vi "CSM - Mermaid - DebugTool.vi"() -> ()   [LabVIEW 2020]
doc: "Show CSM relationship Graph with mermaid"
uses:
  <vilib>/sklein/WebView2 XControl/WebView2 XControl/WebView2 Control.xctl
  <userlib>/_NEVSTOP/Communicable State Machine(CSM)/_Support/Typedef/_CSM_GlobalLog_MSG.ctl
  <userlib>/_NEVSTOP/Communicable State Machine(CSM)/_Support/Typedef/_CSM_Response Source Message.ctl
  <userlib>/_NEVSTOP/Communicable State Machine(CSM)/_Support/Typedef/_CSM_GlobalLog_MSG_TYPE.ctl
  <userlib>/_NEVSTOP/Communicable State Machine(CSM)/AdvanceAPI/CSM - Convert Error to Argument.vi
  <userlib>/_NEVSTOP/Communicable State Machine(CSM)/_Support/GlobalEvent/GEvt-Generate with Rule Check.vi
  <userlib>/_NEVSTOP/Communicable State Machine(CSM)/_Support/GlobalEvent/Cache-GEvt Refs.vi
  <userlib>/_NEVSTOP/Communicable State Machine(CSM)/AdvanceAPI/CSM - Make String Arguments Safe.vi
  <userlib>/_NEVSTOP/Communicable State Machine(CSM)/_Support/ChangeFlag/FlagInstance-GEvt Refs.vi
  <userlib>/_NEVSTOP/Communicable State Machine(CSM)/AdvanceAPI/CSM - Keywords.vi
  <userlib>/_NEVSTOP/Communicable State Machine(CSM)/_Support/ChangeFlag/ChangeFlag-Read.vi
  <userlib>/_NEVSTOP/Communicable State Machine(CSM)/_Polymophic/Add State(s) to Queue By BOOL(Element).vi
  <userlib>/_NEVSTOP/Communicable State Machine(CSM)/_Support/ChangeFlag/ChangeFlagDB.vi
  <userlib>/_NEVSTOP/Communicable State Machine(CSM)/_Support/GlobalEvent/FGV-GlobalEventRef(lvlibp).vi
  <userlib>/_NEVSTOP/Communicable State Machine(CSM)/_Support/GlobalEvent/FGV-GlobalEventQueues(lvlibp).vi
  <userlib>/_NEVSTOP/Communicable State Machine(CSM)/_Support/GlobalEvent/GEvt-Valid Subscribers.vi
  <userlib>/_NEVSTOP/Communicable State Machine(CSM)/_Support/GlobalEvent/LogFilter/LogFilter - Check.vi
  <userlib>/_NEVSTOP/Communicable State Machine(CSM)/_csmHelper/API/Create From VI Reference.vi
  <userlib>/_NEVSTOP/Communicable State Machine(CSM)/_csmHelper/API/Destroy.vi
  <userlib>/_NEVSTOP/Communicable State Machine(CSM)/_Support/GlobalEvent/LogFilter/LogFilter.lvclass
  <userlib>/_NEVSTOP/Communicable State Machine(CSM)/Communicable State Machine.lvlib
  _support/CSM Mermaid Support.lvlib
  <userlib>/_NEVSTOP/Communicable State Machine(CSM)/_csmHelper/CSM-Helper.lvclass
  <userlib>/_NEVSTOP/Communicable State Machine(CSM)/_tool/_file/csm-file-support.lvlib
  <userlib>/_NEVSTOP/Communicable State Machine(CSM)/_tool/_ui/csm-ui-support.lvlib
panel:
  in  "CSM":string(combo)
  in  "Search Button":bool
  in  "Draw Mermaid":bool
  in  "Type":T1(ring)
  in  "Tab":T2(tab)
  out "Broadcast Registry":string[][](table)
  out "mermaid string":string
  in  "WebView2 Control":string(xcontrol)
  # "https://mermaid.live/"
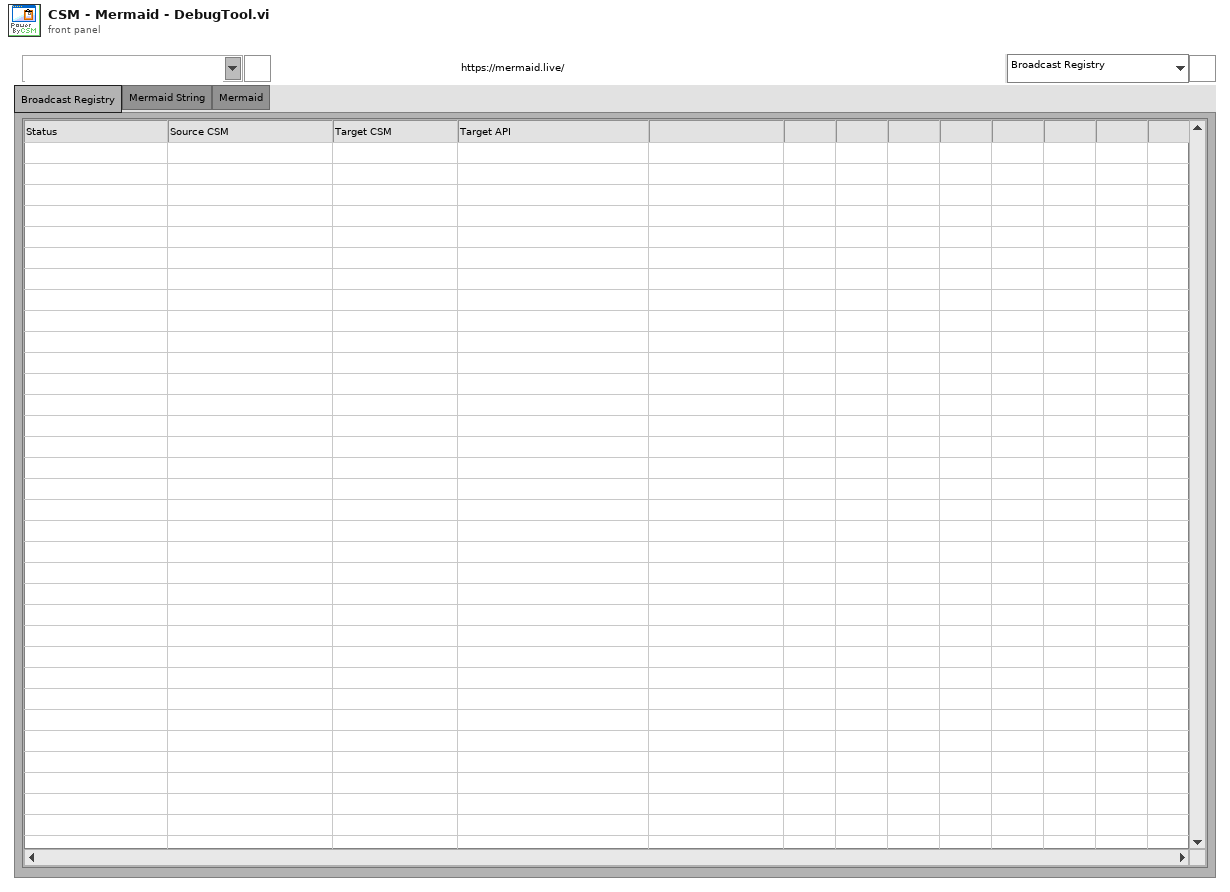
[diagram p1: front panel]
types:
  T1 = enum16{"Broadcast Registry", "CSM Interface", "CSM All Interfaces"}
  T2 = enum32{"Broadcast Registry", "Mermaid String", "Mermaid"}
  T3 = typedef "Communicable State Machine.lvlib/_CSM_GlobalLog_MSG.ctl" = cluster{"Name (\"\" to Use UUID)":string, "Current State":string, "Arguments":string, "Source Message":T4, "Source Module":string, "Complete(T)/Start(F)":bool, "LogType":T5, "Time Stamp":timestamp}
  T4 = typedef "Communicable State Machine.lvlib/_CSM_Response Source Message.ctl" = cluster{"‘State":string, "’Arguments":string, "’Error":errorcluster}
  T5 = typedef "Communicable State Machine.lvlib/_CSM_GlobalLog_MSG_TYPE.ctl" = enum16{"User Log", "State Change", "Status", "Interrupt", "Register", "Unregister", "Error Log", "Module Created", "Module Destroyed", "Async Message", "No-Rep Async Message", "Sync Message"}
  T6 = enum32{"Broadcast Registry", "Mermaid String", "Mermaid", "Error History"}
  T7 = enum32{"Invalid", "Standard", "Closed", "Hidden", "Minimized", "Maximized"}
  T8 = enum32{"invalid app kind", "Development System", "Run Time System", "Student Edition", "Embedded LabVIEW", "Evaluation", "Custom"}
  T9 = cluster{"Shift":bool, "Ctrl":bool, "Alt":bool, "Cmd":bool, "Opt":bool}
  T10 = cluster{"Core":cluster{"Current VI Reference":refnum<vi>, "Close Panel on Exit?":bool}, "Toolbar.Advance":refnum<vi>[], "LoggerWatchDogQueue":refnum<queue>, "LogFile":path, "Mermaid":cluster{"Template":string, "output path":path, "string":string}}
  T11 = cluster{"Template":string, "output path":path, "string":string}
  T12 = cluster{"Current VI Reference":refnum<vi>, "Close Panel on Exit?":bool}
  T13 = cluster{"Status":string, "Source CSM":string, "Target CSM":string, "Target API":string}[]
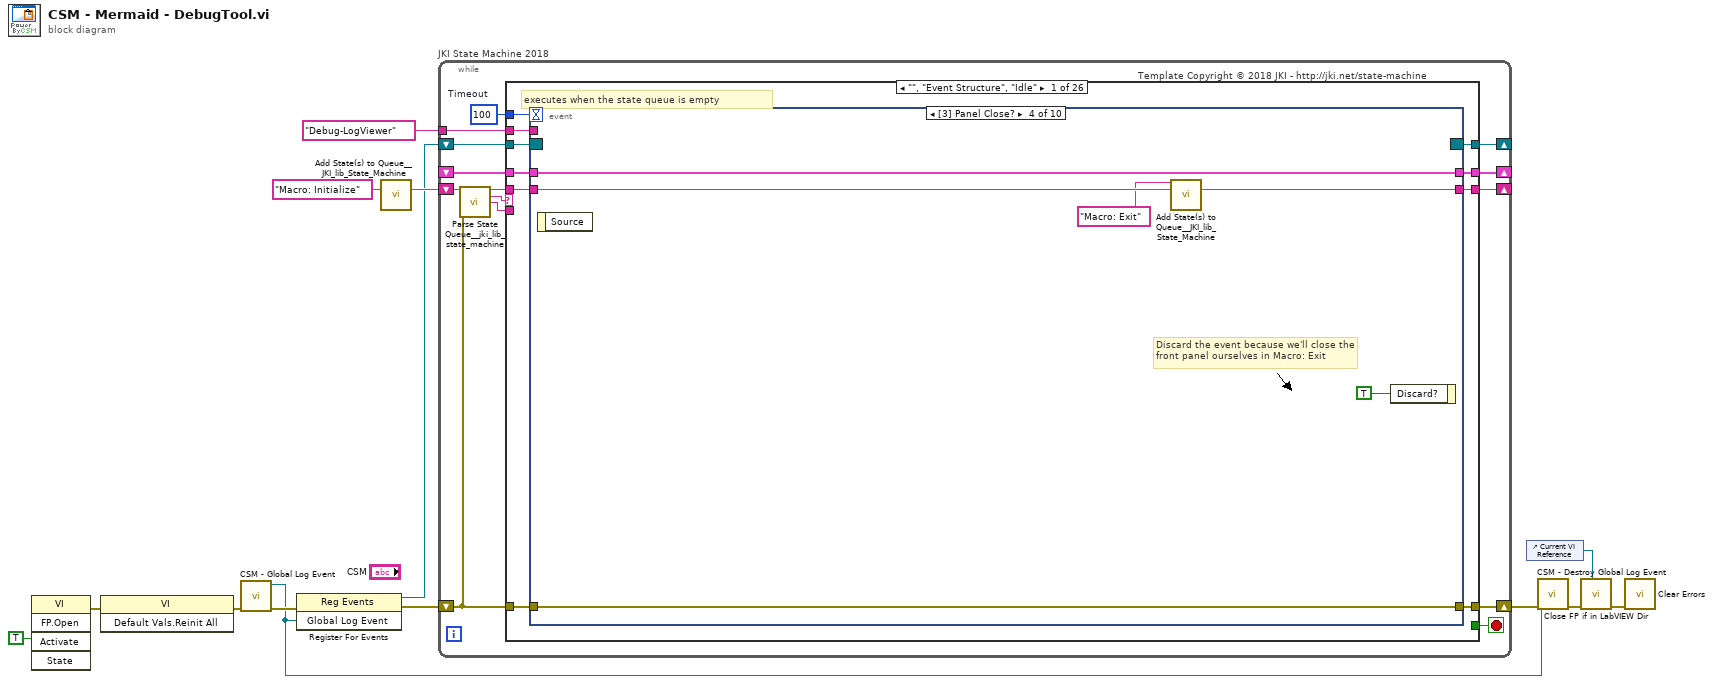
[diagram p0: block diagram]
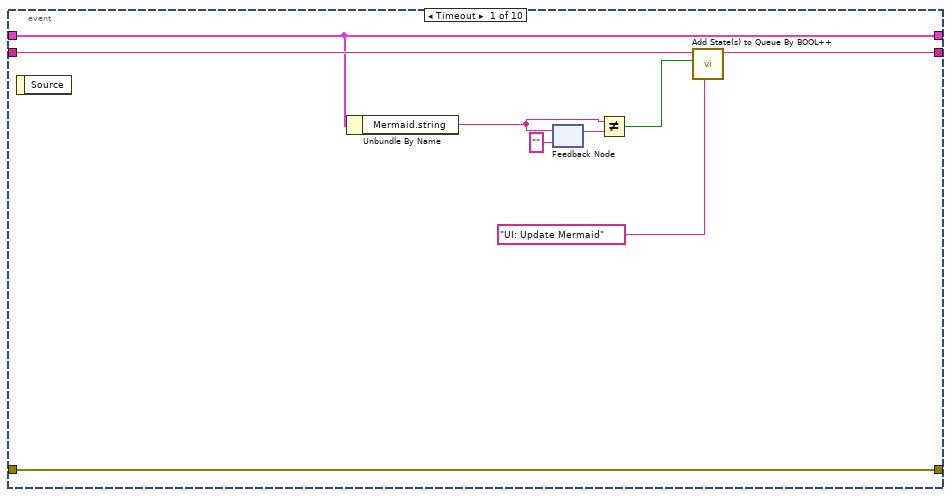
[diagram p2: hidden frame]
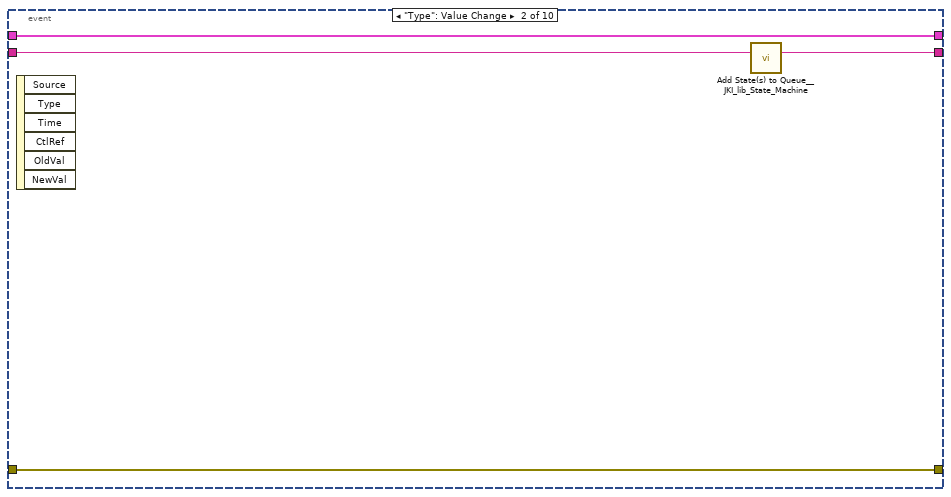
[diagram p3: hidden frame]
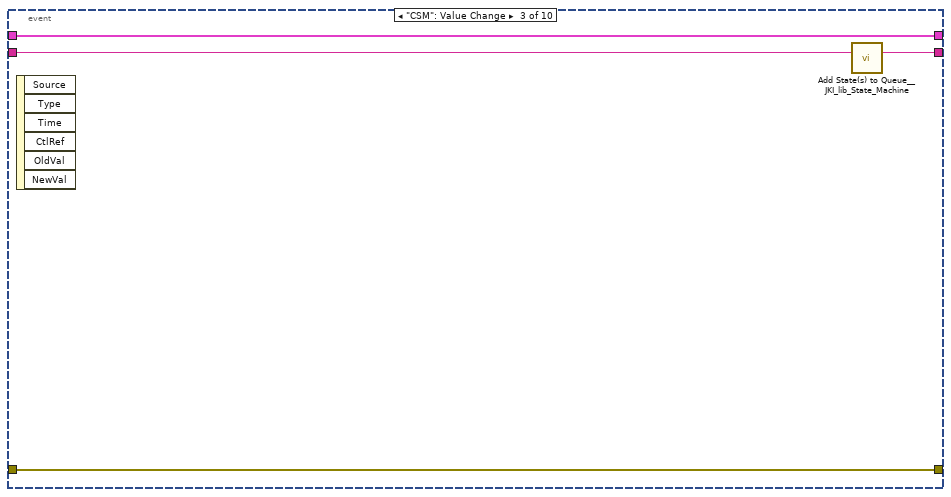
[diagram p4: hidden frame]
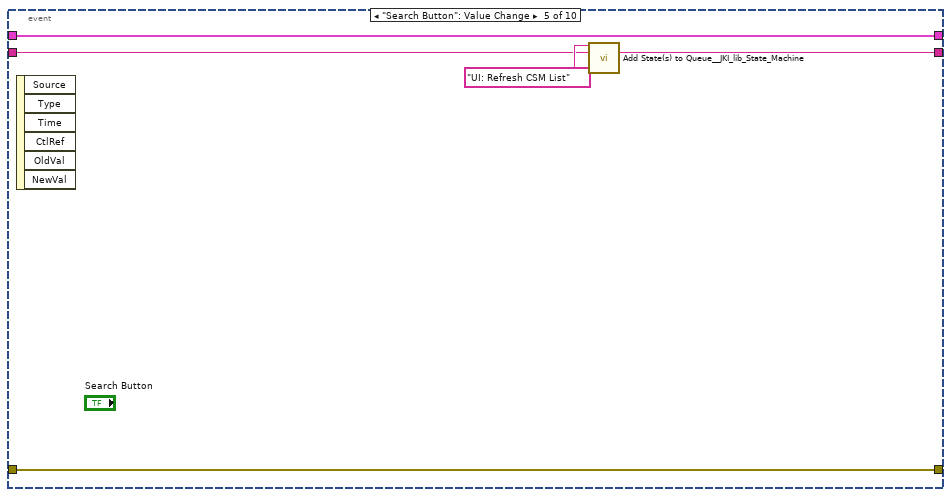
[diagram p5: hidden frame]
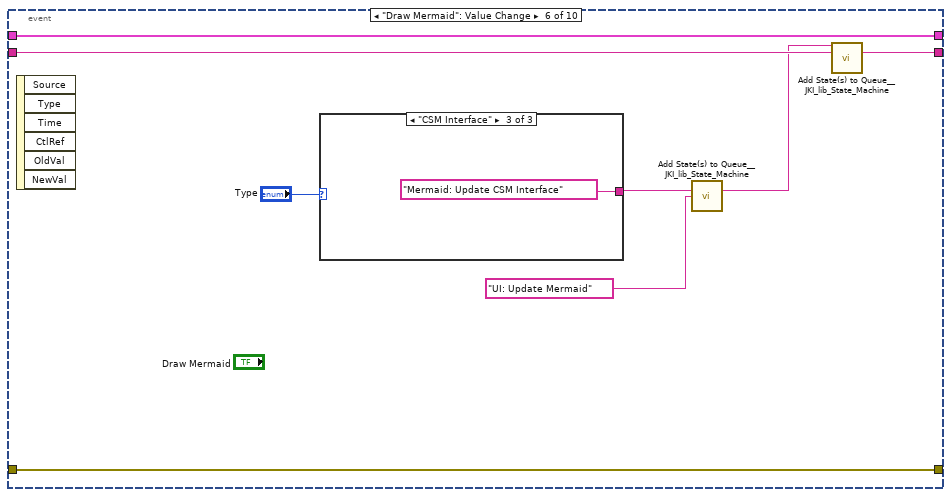
[diagram p6: hidden frame]
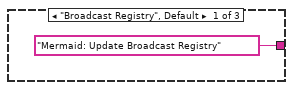
[diagram p7: hidden frame]
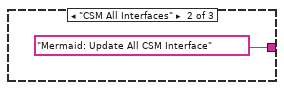
[diagram p8: hidden frame]
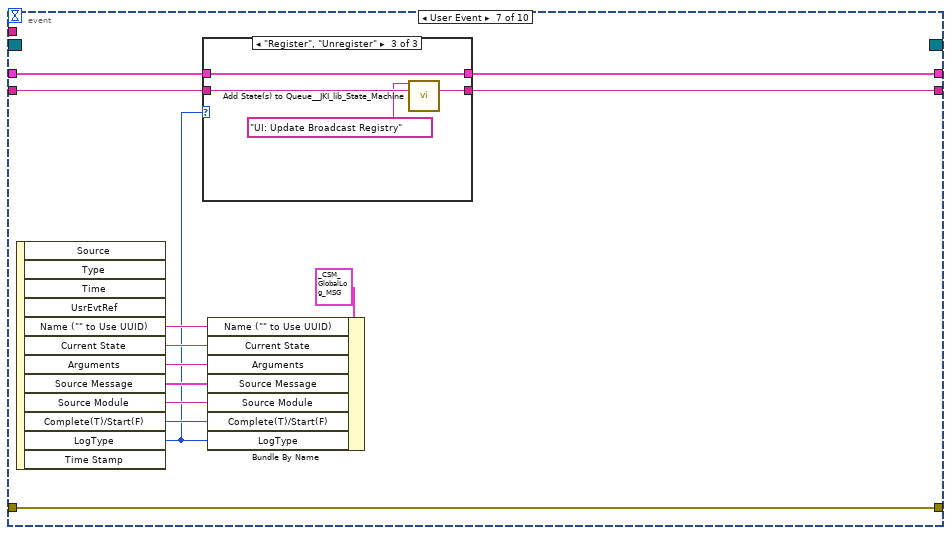
[diagram p9: hidden frame]
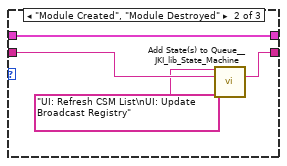
[diagram p11: hidden frame]
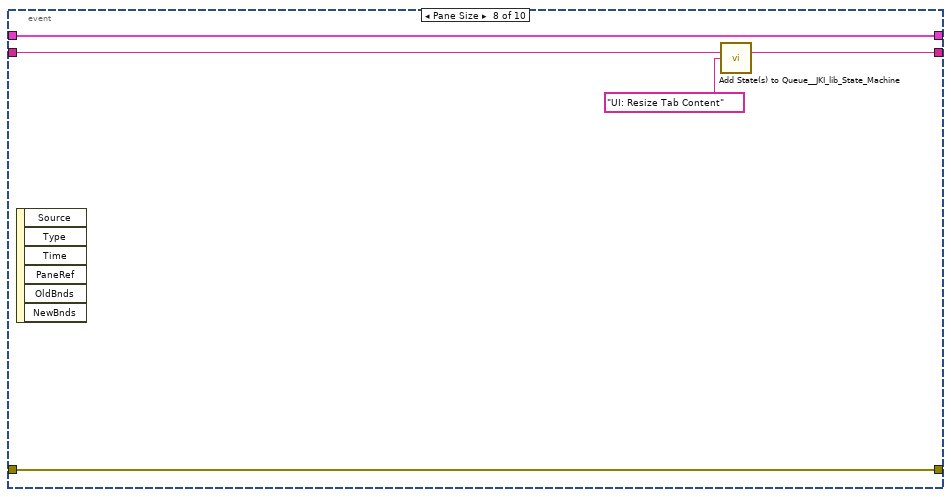
[diagram p12: hidden frame]
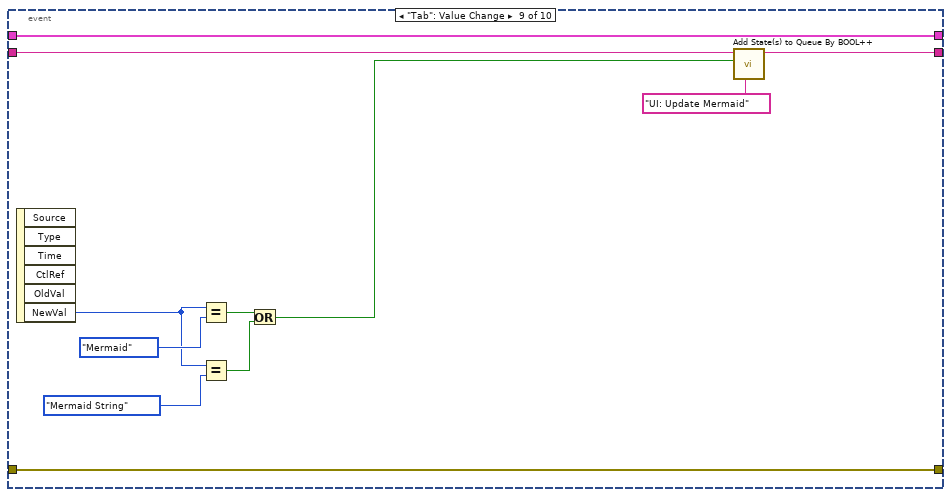
[diagram p13: hidden frame]
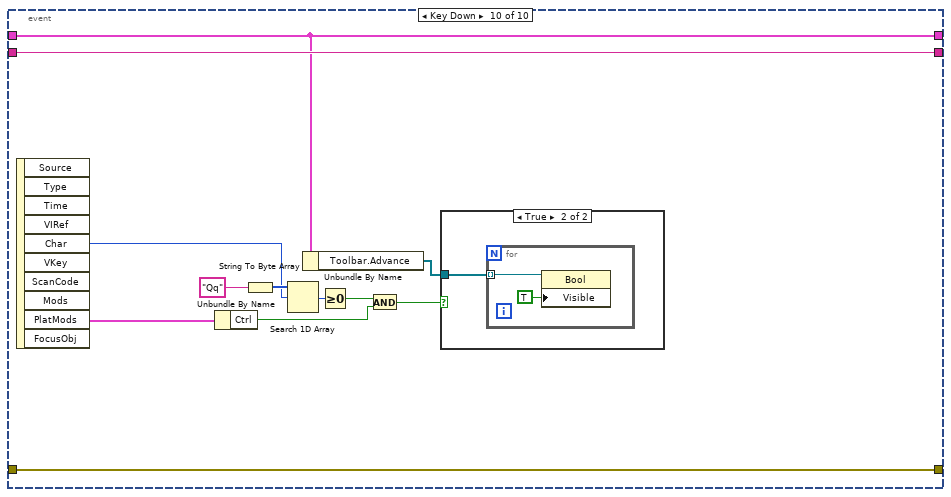
[diagram p14: hidden frame]
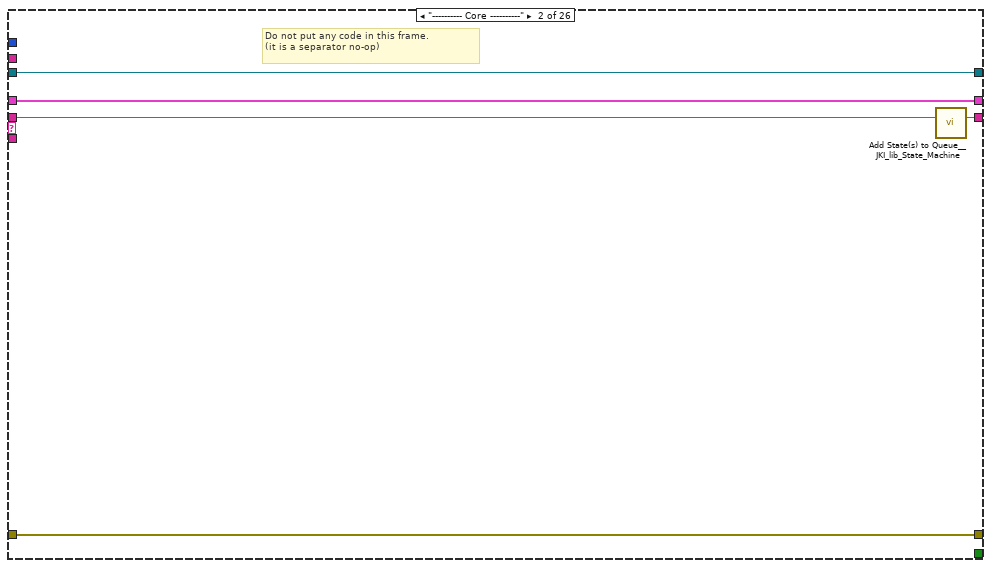
[diagram p16: hidden frame]
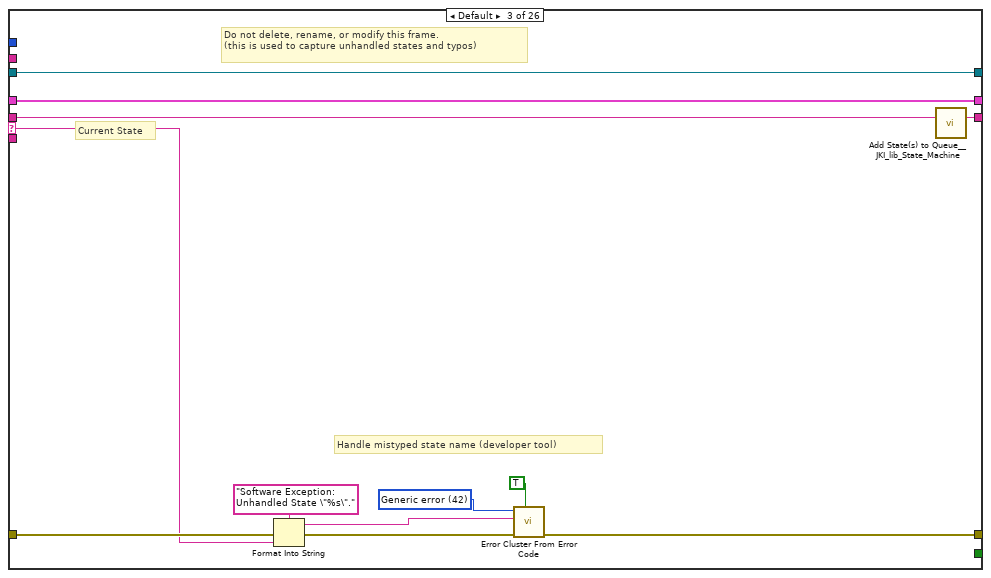
[diagram p17: hidden frame]
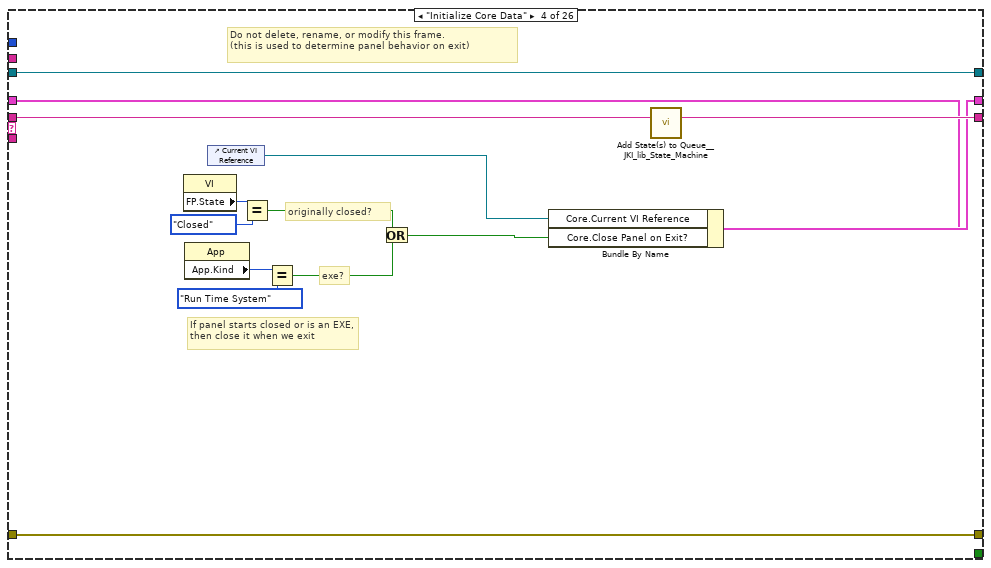
[diagram p18: hidden frame]
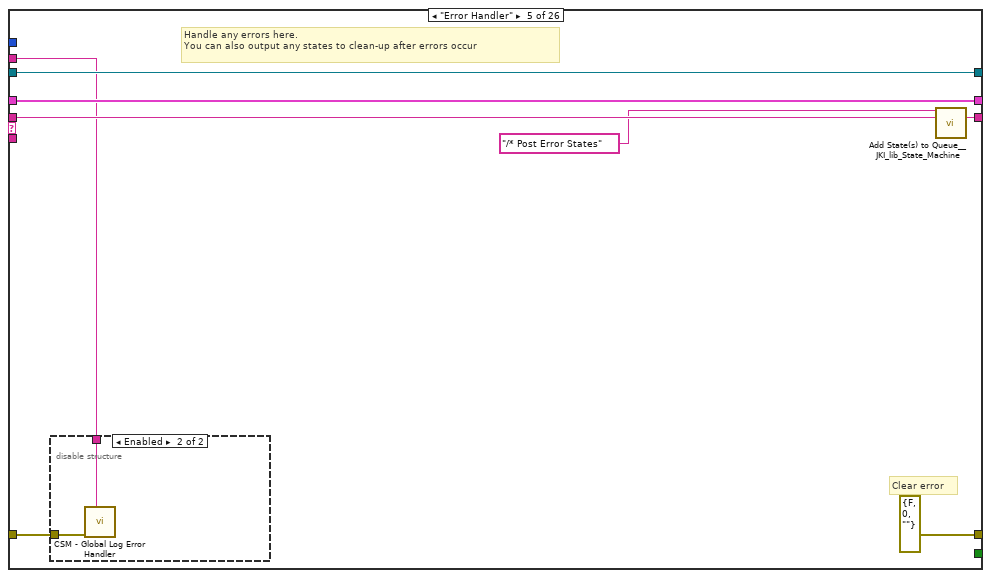
[diagram p19: hidden frame]
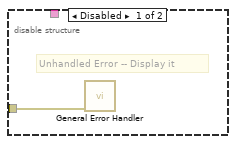
[diagram p20: hidden frame]
diagram:
  n1 = invoke class="VI" method="FP.Open"("Activate"=TRUE ("Activate?")) -> (error out=w13:errorcluster)  [unwired: 4 in, 4 out]
  n2 = invoke class="VI" method="Default Vals.Reinit All"(error in=w13) -> (error out=w8:errorcluster)  [unwired: 2 in, 2 out]
  n3 = call <userlib>:"CSM - Global Log Event.vi"("Error In"=w8) -> ("error out"=w12:errorcluster, "Global Log Event"=w11:refnum<user-event>)  [unwired: 9 in]
  n4 = register-events(error in=w12, w11) -> (reference out=w6:refnum<event-registration>, error out=w7:errorcluster)  [unwired: 1 in]
  n5 = call <vilib>:"Add State(s) to Queue__JKI_lib_State_Machine.vi"("State(s) in (\"\")"="Macro: Initialize") -> ("States Out"=w10:string)  [unwired: 14 in]
  n6 = while "JKI State Machine 2018" {
    shift-right: [w21] -> _
    shift-left: _ -> [w20]
    shift-right: [w24] -> w5
    shift-left: w7 -> [w18]
    shift-right: [w23] -> _
    shift-left: w10 -> [w25]
    shift-right: [w16] -> _
    shift-left: w6 -> [w17]
    tunnel: "Debug-LogViewer" ("Current Module(\"\" to generate a ID)") -> [w15]
    stop <- w22 stop-if-true
    w19 = 100  # Timeout
    # "Template Copyright © 2018 JKI - http://jki.net/state-machine"
    n7 = call <vilib>:"Parse State Queue__jki_lib_state_machine.vi"("State Queue"=w25, "Error In (no error)"=w18) -> ("Remaining States"=w27:string, "Current State"=w28:string, "Arguments"=w26:string)  [unwired: 11 in]
    n8 = case shown="\"\", \"Event Structure\", \"Idle\"" w28 {
      selector: w28 -> [_ _ w138 _ _ _ _ _ _ _ _ _ _ _ _ _ _ _ _ _ _ _ _ _ _ _]
      tunnel: w27 -> [w38 w136 w142 w162 w170 w179 w184 w211 w221 w229 w234 w239 w248 w260 w335 w338 w358 w375 w399 w410 w416 w432 w439 w442 w460 w491]
      tunnel: w26 -> [_ _ _ _ _ _ _ _ _ _ _ _ w243 w254 _ _ _ _ _ _ _ _ _ _ _ _]
      tunnel: w20 -> [w36 w133 w140 w155 w167 w174 w181 _ w220 w224 w231 w236 w246 w256 w334 w342 w356 w373 w398 w407 w413 w417 w438 w446 w459 w490]
      tunnel: [w35 w134 w144 w159 errorcluster {"status"=FALSE, "code"=0, "source"=""} ("error out") w177 w182 w208 w218 w222 w232 _ w244 w257 w336 w343 w359 w376 w400 w408 w414 w430 w440 w447 w448 w481] -> w24
      tunnel: w18 -> [w34 w134 w143 w159 w166 w177 w182 w208 w218 w226 w232 _ w245 w258 w336 w343 w359 w376 w400 w408 w414 w430 w440 w447 w448 w481]
      tunnel: [w37 w135 w141 w161 w169 w178 w183 w210 w221 w228 w233 w238 w247 w259 w335 w339 w358 w375 w399 w409 w415 w431 w439 w443 w460 w491] -> w23
      tunnel: [_ _ _ _ _ TRUE _ _ _ _ _ _ _ _ _ _ _ _ _ _ _ _ _ _ _ _] -> w22
      tunnel: [w33 w133 w140 w160 w167 w174 w181 w195 w220 w224 w231 w236 w246 w256 w334 w342 w356 w373 w398 w407 w413 w417 w438 w444 w457 w488] -> w21
      tunnel: w19 -> [w32 _ _ _ _ _ _ _ _ _ _ _ _ _ _ _ _ _ _ _ _ _ _ _ _ _]
      tunnel: w17 -> [w31 w132 w137 w149 w164 w175 w180 w206 w219 w223 w230 w237 w242 w253 w333 w341 w357 w374 w397 w406 w411 w423 w437 w445 w458 w489]
      tunnel: [w30 w132 w137 w149 w164 w175 w180 w206 w219 w223 w230 w237 w242 w253 w333 w341 w357 w374 w397 w406 w411 w423 w437 w445 w458 w489] -> w16
      tunnel: w15 -> [w29 _ _ _ w163 _ _ _ _ _ _ _ _ _ _ _ _ _ _ _ _ _ _ _ w455 w486]
      frame "", "Event Structure", "Idle" {
        # "executes when the state queue is empty"
        n9 = event shown="[3] Panel Close?" {
          selector: w31 -> [_ _ _ _ _ _ _ _ _ _]
          dyn-events: [_ _ _ _ _ _ _ _ _ _] -> w30
          timeout: w32 -> [_ _ _ _ _ _ _ _ _ _]
          tunnel: w38 -> [w47 w48 w52 w61 w63 w70 w82 w102 w113 w128]
          tunnel: [w46 w49 w53 w60 w62 w71 w81 w103 w114 w128] -> w37
          tunnel: w36 -> [w43 w50 w54 w58 w66 w73 w78 w104 w115 w119]
          tunnel: [w45 w51 w55 w59 w65 w74 w90 w105 w116 w127] -> w35
          tunnel: w34 -> [w45 w51 w55 w59 w65 w74 w90 w105 w116 w127]
          tunnel: [w43 w50 w54 w58 w66 w73 w79 w104 w115 w119] -> w33
          tunnel: w29 -> [_ _ _ _ _ _ _ _ _ _]
          event Timeout {
            n10 = event-data() -> ()  [unwired: 1 in, 1 out]
            n11 = Unbundle By Name(w43) -> ("Mermaid.string"=w40:string)
            n12 = feedback #1("" ("string")) -> (w41:string)
            n13 = feedback-in #1(w40) -> ()
            n14 = Not Equal?(x=w40, y=w41) -> (x != y?=w39:bool)
            n15 = call-poly <userlib>:"Add State(s) to Queue By BOOL++.vi"("TRUE (\"\")"="UI: Update Mermaid" ("State(s) in Front (\"\")"), "Condition"=w39, "State Queue (\"\")"=w47) -> ("Remaining States"=w46:string)  [unwired: 8 in]
          }
          event "Type": Value Change {
            n16 = event-data() -> ()  [unwired: 1 in, 6 out]
            n17 = call <vilib>:"Add State(s) to Queue__JKI_lib_State_Machine.vi"("State(s) in (\"\")"=w48) -> ("States Out"=w49:string)  [unwired: 14 in]
          }
          event "CSM": Value Change {
            n18 = event-data() -> ()  [unwired: 1 in, 6 out]
            n19 = call <vilib>:"Add State(s) to Queue__JKI_lib_State_Machine.vi"("State(s) in (\"\")"=w52) -> ("States Out"=w53:string)  [unwired: 14 in]
          }
          event Panel Close? {
            # "Discard the event because we'll close the front panel ourselves in Macro: Exit"
            n20 = event-data() -> ()  [unwired: 1 in, 1 out]
            n21 = call <vilib>:"Add State(s) to Queue__JKI_lib_State_Machine.vi"("State(s) in Front (\"\")"="Macro: Exit", "State(s) in (\"\")"=w61) -> ("States Out"=w60:string)  [unwired: 13 in]
            n22 = event-data("Discard?"=TRUE) -> ()  [unwired: 1 in, 1 out]
          }
          event "Search Button": Value Change {
            n23 = event-data() -> ()  [unwired: 1 in, 6 out]
            n24 = call <vilib>:"Add State(s) to Queue__JKI_lib_State_Machine.vi"("State(s) in Front (\"\")"="UI: Refresh CSM List" ("State(s) in Front (\"\")"), "State(s) in (\"\")"=w63) -> ("States Out"=w62:string)  [unwired: 13 in]
          }
          event "Draw Mermaid": Value Change {
            n25 = event-data() -> ()  [unwired: 1 in, 6 out]
            n26 = case shown="\"CSM Interface\"" "Type" {
              tunnel: ["Mermaid: Update Broadcast Registry" ("State(s) in Front (\"\")") "Mermaid: Update All CSM Interface" ("State(s) in Front (\"\")") "Mermaid: Update CSM Interface" ("State(s) in Front (\"\")")] -> w69
              frame "Broadcast Registry", Default {
              }
              frame "CSM All Interfaces" {
              }
              frame "CSM Interface" {
              }
            }
            n27 = call <vilib>:"Add State(s) to Queue__JKI_lib_State_Machine.vi"("State(s) in (\"\")"=w69, "State(s) at Back (\"\")"="UI: Update Mermaid" ("State(s) in Front (\"\")")) -> ("States Out"=w67:string)  [unwired: 13 in]
            n28 = call <vilib>:"Add State(s) to Queue__JKI_lib_State_Machine.vi"("State(s) in Front (\"\")"=w67, "State(s) in (\"\")"=w70) -> ("States Out"=w71:string)  [unwired: 13 in]
          }
          event User Event {
            n29 = event-data() -> ("Name (\"\" to Use UUID)"=w88:string, "Current State"=w87:string, "Arguments"=w86:string, "Source Message"=w85:T4, "Source Module"=w84:string, "Complete(T)/Start(F)"=w83:bool, "LogType"=w80:T5)  [unwired: 1 in, 5 out]
            n30 = case shown="\"Register\", \"Unregister\"" w80 {
              tunnel: w82 -> [w92 w96 w100]
              tunnel: [w92 w95 w99] -> w81
              tunnel: [w91 w93 w97] -> w79
              tunnel: w78 -> [w91 w93 w97]
              frame "User Log", Default {
              }
              frame "Module Created", "Module Destroyed" {
                n31 = call <vilib>:"Add State(s) to Queue__JKI_lib_State_Machine.vi"("State(s) in Front (\"\")"="UI: Refresh CSM List\nUI: Update Broadcast Registry" ("State(s) in Front (\"\")"), "State(s) in (\"\")"=w96) -> ("States Out"=w95:string)  [unwired: 13 in]
              }
              frame "Register", "Unregister" {
                n32 = call <vilib>:"Add State(s) to Queue__JKI_lib_State_Machine.vi"("State(s) in Front (\"\")"="UI: Update Broadcast Registry" ("State(s) in Front (\"\")"), "State(s) in (\"\")"=w100) -> ("States Out"=w99:string)  [unwired: 13 in]
              }
            }
            n33 = Bundle By Name(cluster=T3 {"Name (\"\" to Use UUID)"="", "Current State"="", "Arguments"="", "Source Message"={"‘State"="", "’Arguments"="", "’Error"={"status"=FALSE, "code"=0, "source"=""}}, "Source Module"="", "Complete(T)/Start(F)"=FALSE, "LogType"=enum."State Change", "Time Stamp"=timestamp(0 s since 1904-01-01)} ("Cross CSM Data"), "Name (\"\" to Use UUID)"=w88, "Current State"=w87, "Arguments"=w86, "Source Message"=w85, "Source Module"=w84, "Complete(T)/Start(F)"=w83, "LogType"=w80) -> ()  [unwired: 1 out]
          }
          event Pane Size {
            n34 = event-data() -> ()  [unwired: 1 in, 6 out]
            n35 = call <vilib>:"Add State(s) to Queue__JKI_lib_State_Machine.vi"("State(s) in (\"\")"=w102, "State(s) at Back (\"\")"="UI: Resize Tab Content" ("State(s) in Front (\"\")")) -> ("States Out"=w103:string)  [unwired: 13 in]
          }
          event "Tab": Value Change {
            n36 = event-data() -> ("NewVal"=w107:T2)  [unwired: 1 in, 5 out]
            n37 = Equal?(x=w107, y=T6."Mermaid") -> (x = y?=w110:bool)
            n38 = Equal?(x=w107, y=T6."Mermaid String") -> (x = y?=w106:bool)
            n39 = Or(x=w110, y=w106) -> (x .or. y?=w109:bool)
            n40 = call-poly <userlib>:"Add State(s) to Queue By BOOL++.vi"("TRUE (\"\")"="UI: Update Mermaid" ("TRUE(\"\")"), "Condition"=w109, "State Queue (\"\")"=w113) -> ("Remaining States"=w114:string)  [unwired: 8 in]
          }
          event Key Down {
            n41 = event-data() -> ("Char"=w117:i16, "PlatMods"=w122:T9)  [unwired: 1 in, 8 out]
            n42 = Unbundle By Name(w122) -> ("Ctrl"=w121:bool)
            n43 = String To Byte Array(string="Qq") -> (unsigned byte array=w124:u8[])
            n44 = Search 1D Array(1D array=w124, element=w117) -> (index of element=w125:i32)  [unwired: 1 in]
            n45 = Unbundle By Name(w119) -> ("Toolbar.Advance"=w118:refnum<vi>[])
            n46 = Greater Or Equal To 0?(x=w125) -> (x >= 0?=w126:bool)
            n47 = And(x=w126, y=w121) -> (x .and. y?=w120:bool)
            n48 = case shown="True" w120 {
              tunnel: w118 -> [_ w129]
              frame False {
              }
              frame True {
                n49 = for {
                  tunnel: w129 -> [w131] mode=indexing
                  n50 = property class="Bool"(reference=w131, "Visible"=TRUE) -> ()  [unwired: 1 in, 2 out]
                }
              }
            }
          }
        }
      }
      frame "---------- Core ----------" {
        # "Do not put any code in this frame.\n(it is a separator no-op)"
        n51 = call <vilib>:"Add State(s) to Queue__JKI_lib_State_Machine.vi"("State(s) in (\"\")"=w136) -> ("States Out"=w135:string)  [unwired: 14 in]
      }
      frame Default {
        w147 = 42 items=["No error", "Argument error", "Memory is full", "Out of zone", "End of file", "File already open", "Generic file I/O error", "File not found", "File permission error", "Disk is full", "Duplicate path", "Too many files open", "System feature not enabled", "Resource file not found", "Cannot add resource", "Resource not found", "Image not found", "Image memory error", "Pen does not exist", "Config type invalid", "Config token not found", "Config parse error", "Config memory error", "Bad external code format", "Bad external code offset", "External code not present", "Null window", "Destroy window error", "Null menu", "Print aborted", "Bad print record", "Print driver error", "Windows error during printing", "Memory error during printing", "Print dialog error", "Generic print error", "Invalid device refnum", "Device not found", "Device parameter error", "Device unit error", "Cannot open device", "Device call aborted", "Generic error", "Cancelled by user", "Object ID too low", "Object ID too high", "Object not in heap", "Unknown heap", "Unknown object (invalid DefProc)", "Unknown object (DefProc not in table)", "Message out of range", "Invalid (null) method", "Unknown message", "Manager call not supported", "Bad address", "Network operation in progress", "Network operation timed out", "Connection is busy", "Network attribute not supported", "Network error", "Address in use", "System out of memory", "Connection aborted", "Connection refused", "Not connected", "Already connected", "Connection closed", "Initialization error (interapplication manager)", "Bad occurrence", "Wait on unbound occurrence handler", "Occurrence queue overflow", "Datalog type conflict", "Unused", "Unrecognized type (interapplication manager)", "Memory corrupt", "Failed to make temporary DLL", "Old CIN version", "Drag socket not found", "Failed to load drop-object", "Failed to register OLE object", "Failed to release OLE object", "Format specifier type mismatch", "Unknown format specifier", "Too few format specifiers", "Too many format specifiers", "Scan failed", "Newer CIN version", "Error converting to variant", "Runtime menu error", "Password tampered", "Variant attribute not found", "Incompatible variant data type", "Event data is not available", "Event Store is not present", "Occurrence is not found", "Event Queue is not created", "Event info is not available", "Refnum passed is NULL", "Error retrieving Class GUID", "Error retrieving CoClass GUID", "Error retrieving TypeLib GUID.", "Bad built application magic bytes.", "Specific driver is different from the specific driver associated with the Logical Name.", "There is no session opened to the class driver.", "Max Error", "MAX - Error with config objects", "MAX - Error loading configuration", "MAX - Group not supported"]
        # "Current State"
        # "Do not delete, rename, or modify this frame.\n(this is used to capture unhandled states and typos)"
        # "Handle mistyped state name (developer tool)"
        n52 = Format Into String(format string="Software Exception: Unhandled State \"%s\"." ("message"), error in=w143, w138) -> (resulting string=w146:string, error out=w145:errorcluster)  [unwired: 1 in]
        n53 = call <vilib>:"Error Cluster From Error Code.vi"("show call chain? (False)"=TRUE, "error in (no error)"=w145, "error message (\"\")"=w146, "error code (0)"=w147) -> ("error out"=w144:errorcluster)  [unwired: 5 in]
        n54 = call <vilib>:"Add State(s) to Queue__JKI_lib_State_Machine.vi"("State(s) in (\"\")"=w142) -> ("States Out"=w141:string)  [unwired: 14 in]
      }
      frame "Initialize Core Data" {
        # "Do not delete, rename, or modify this frame.\n(this is used to determine panel behavior on exit)"
        # "originally closed?"
        # "exe?"
        # "If panel starts closed or is an EXE, then close it when we exit"
        n55 = property class="VI"() -> ("FP.State"=w152:T7)  [unwired: 2 in, 2 out]
        n56 = property class="App"() -> ("App.Kind"=w158:T8)  [unwired: 2 in, 2 out]
        n57 = control-ref of="Current VI Reference"() -> (w153:refnum<vi>)
        n58 = Equal?(x=w152, y=T7."Closed" ("Front Panel Window:State")) -> (x = y?=w150:bool)
        n59 = Equal?(x=w158, y=T8."Run Time System" ("Application:Kind")) -> (x = y?=w156:bool)
        n60 = Or(x=w150, y=w156) -> (x .or. y?=w154:bool)
        n61 = Bundle By Name(cluster=w155, "Core.Current VI Reference"=w153, "Core.Close Panel on Exit?"=w154) -> (w160:T10)
        n62 = call <vilib>:"Add State(s) to Queue__JKI_lib_State_Machine.vi"("State(s) in (\"\")"=w162) -> ("States Out"=w161:string)  [unwired: 14 in]
      }
      frame "Error Handler" {
        # "Handle any errors here.\nYou can also output any states to clean-up after errors occur"
        # "Clear error"
        n63 = disable-structure "Diagram Disable Structure" shown="Enabled" {
          disable-tunnel: w166 -> [w171 w173]
          disable-tunnel: w163 -> [_ w172]
          frame Disabled {
            # "Unhandled Error -- Display it"
            n64 = call <vilib>:"General Error Handler.vi"("error in (no error)"=w171) -> ()  [unwired: 10 in, 5 out]
          }
          frame Enabled {
            n65 = call <userlib>:"CSM - Global Log Error Handler.vi"("Place (\"\" to Use VI's Name)"=w172, "Error In"=w173) -> ()  [unwired: 9 in, 1 out]
          }
        }
        n66 = call <vilib>:"Add State(s) to Queue__JKI_lib_State_Machine.vi"("State(s) in Front (\"\")"="/* Post Error States", "State(s) in (\"\")"=w170) -> ("States Out"=w169:string)  [unwired: 13 in]
      }
      frame "Exit" {
        # "Do not put any code in this frame.\n(No errors that occur here will be handled.)"
        n67 = call <vilib>:"Add State(s) to Queue__JKI_lib_State_Machine.vi"("State(s) in (\"\")"=w179) -> ("States Out"=w178:string)  [unwired: 14 in]
      }
      frame "---------- Data ----------" {
        # "Do not put any code in this frame.\n(It is a separator no-op. You can make a copy of this frame to create a new Data frame)"
        n68 = call <vilib>:"Add State(s) to Queue__JKI_lib_State_Machine.vi"("State(s) in (\"\")"=w184) -> ("States Out"=w183:string)  [unwired: 14 in]
      }
      frame "Data: Initialize" {
        w196 = T11 {"Template"="", "output path"=path "", "string"=""}  # Mermaid
        w203 = path ""  # LogFile
        w204 = refnum<queue> refnum  # LoggerWatchDogQueue
        w205 = refnum<vi>[] []  # Toolbar.Advance
        w207 = T12 {"Current VI Reference"=refnum, "Close Panel on Exit?"=FALSE}  # Core
        # "Initialize the shift-register data, here.\n(data names are defined by what you wire into the bundle function)"
        n69 = control-ref of="Current VI Reference"() -> (w193:refnum<vi>)
        n70 = property class="VI"(reference=w193) -> (reference out=w191:refnum<vi>, "VI Path"=w192:path)  [unwired: 1 in, 1 out]
        n71 = Close Reference(reference=w191) -> ()  [unwired: 1 in, 1 out]
        n72 = while {
          shift-right: [w212] -> w190
          shift-left: w192 -> [w214]
          stop <- w216 stop-if-true
          # "is Dir?"
          n73 = Strip Path(path=w214) -> (stripped path=w212:path)  [unwired: 1 out]
          n74 = File/Directory Info(path=w212) -> (directory=w217:bool)  [unwired: 1 in, 6 out]
          n75 = Not A Number/Path/Refnum?(number/path/refnum=w214) -> (NaN/Path/Refnum?=w215:bool)
          n76 = Empty String/Path?(string/path=w214) -> (empty?=w213:bool)
          n77 = Compound Arithmetic op=OR(w217, w215, w213) -> (w216:bool)
        }
        n78 = Build Path(base path=w190, name or relative path=path "" ("Relative path (.)")) -> (appended path=w188:path)
        n79 = call <vilib>:"Recursive File List.vi"("pattern"="Broadcast Registry Mermaid.html" ("pattern(ini by default)"), "Continue Recursing on Error? (F)"=TRUE ("Recrusively(F)"), "Folder Path"=w188) -> ("All Files in Dir"=w187:path[])  [unwired: 4 in, 4 out]
        n80 = Index Array(array=w187) -> (element=w186:path)  [unwired: 1 in]
        n81 = call <userlib>:"uuid.vi"() -> ("UUID"=w197:string)  [unwired: 11 in]
        n82 = Strip Path(path=w186) -> (stripped path=w198:path)  [unwired: 1 out]
        n83 = call <userlib>:"TxtFile Load_CSM.vi"("Path"=w186) -> ("Text"=w185:string)  [unwired: 9 in, 1 out]
        n84 = Concatenate Strings(w197, ".html" ("string")) -> (w199:string)
        n85 = Build Path(base path=w198, name or relative path=w199) -> (appended path=w194:path)
        n86 = Bundle("Core"=w207, "Toolbar.Advance"=w205, "LoggerWatchDogQueue"=w204, "LogFile"=w203, "Mermaid"=w196) -> (w209:T10)  [unwired: 1 in]
        n87 = Bundle By Name(cluster=w209, "Mermaid.Template"=w185, "Mermaid.output path"=w194) -> (w195:T10)
        n88 = call <vilib>:"Add State(s) to Queue__JKI_lib_State_Machine.vi"("State(s) in (\"\")"=w211) -> ("States Out"=w210:string)  [unwired: 14 in]
      }
      frame "Data: Initialize References" {
      }
      frame "Data: Cleanup" {
        # "Cleanup any data and references, here.\n(this is called automatically, by the Macro: Exit)"
        n89 = Unbundle By Name(w224) -> ("Core.Current VI Reference"=w227:refnum<vi>)
        n90 = Close Reference(reference=w227, error in (no error)=w226) -> (error out=w225:errorcluster)
        n91 = Merge Errors(w225) -> (w222:errorcluster)
        n92 = call <vilib>:"Add State(s) to Queue__JKI_lib_State_Machine.vi"("State(s) in (\"\")"=w229) -> ("States Out"=w228:string)  [unwired: 14 in]
      }
      frame "---------- UI ----------" {
        # "Do not put any code in this frame.\n(It is a separator no-op. You can make a copy of this frame to create a new UI frame)"
        n93 = call <vilib>:"Add State(s) to Queue__JKI_lib_State_Machine.vi"("State(s) in (\"\")"=w234) -> ("States Out"=w233:string)  [unwired: 14 in]
      }
      frame "UI: Initialize" {
        # "Initialize the User Interface, here.\n(this is called automatically, by the Macro: Init)"
        n94 = Unbundle By Name(w236) -> ("Toolbar.Advance"=w235:refnum<vi>[])
        n95 = for {
          tunnel: w235 -> [w241] mode=indexing
          n96 = property class="Bool"(reference=w241, "Visible"=FALSE) -> ()  [unwired: 1 in, 2 out]
        }
        n97 = call <vilib>:"Add State(s) to Queue__JKI_lib_State_Machine.vi"("State(s) in (\"\")"=w239) -> ("States Out"=w238:string)  [unwired: 14 in]
      }
      frame "UI: Cursor Set" {
        # "Argument"
        # "Set and Unset Cursor Busy.\n(Usage: \"UI: Cursor Set >> Busy|Idle\")"
        n98 = case shown="\"Idle\", Default" w243 {
          tunnel: w245 -> [w250 w252]
          tunnel: [w249 w251] -> w244
          frame "Idle", Default {
            n99 = call <vilib>:"Unset Busy.vi"("error in (no error)"=w250) -> ("error out"=w249:errorcluster)  [unwired: 10 in]
          }
          frame "Busy" {
            n100 = call <vilib>:"Set Busy.vi"("error in (no error)"=w252) -> ("error out"=w251:errorcluster)  [unwired: 9 in, 1 out]
          }
        }
        n101 = call <vilib>:"Add State(s) to Queue__JKI_lib_State_Machine.vi"("State(s) in (\"\")"=w248) -> ("States Out"=w247:string)  [unwired: 14 in]
      }
      frame "UI: Front Panel State" {
        # "Argument"
        # "Set Front Panel Open or Closed\n(Usage: \"UI: Front Panel State >> Open|Close\")"
        n102 = Unbundle By Name(w256) -> ("Core.Current VI Reference"=w255:refnum<vi>)
        n103 = case shown="\"Minimize\", \"Minimized\"" w254 {
          tunnel: w258 -> [w266 w281 w292 w305 w318]
          tunnel: [w268 w282 w294 w307 w320] -> w257
          tunnel: w255 -> [w267 w279 w293 w306 w319]
          frame "Open", "Standard", Default {
            w261 = T7."Standard" ("State")
            n104 = property class="VI"(reference=w267, error in=w266) -> (reference out=w264:refnum<vi>, error out=w265:errorcluster, "FP.State"=w263:T7)
            n105 = Not Equal?(x=w263, y=w261) -> (x != y?=w262:bool)
            n106 = case shown="True" w262 {
              tunnel: [w272 w274] -> w268
              tunnel: w265 -> [w271 w274]
              tunnel: w264 -> [w270 _]
              tunnel: w261 -> [w269 _]
              frame True {
                n107 = invoke class="VI" method="FP.Open"(reference=w270, error in=w271, "Activate"=TRUE, "State"=w269) -> (error out=w272:errorcluster)  [unwired: 1 in, 4 out]
              }
              frame False {
              }
            }
          }
          frame "Close", "Closed" {
            n108 = property class="VI"(reference=w279, error in=w281) -> (reference out=w278:refnum<vi>, error out=w280:errorcluster, "FP.State"=w276:T7)
            n109 = Not Equal?(x=w276, y=T7."Closed" ("Front Panel Window:State")) -> (x != y?=w275:bool)
            n110 = case shown="True" w275 {
              tunnel: [w283 w286] -> w282
              tunnel: w280 -> [w283 w285]
              tunnel: w278 -> [_ w284]
              frame False {
              }
              frame True {
                n111 = invoke class="VI" method="FP.Close"(reference=w284, error in=w285) -> (error out=w286:errorcluster)  [unwired: 1 in, 2 out]
              }
            }
          }
          frame "Hidden", "Hide" {
            w287 = T7."Hidden" ("State")
            n112 = property class="VI"(reference=w293, error in=w292) -> (reference out=w290:refnum<vi>, error out=w291:errorcluster, "FP.State"=w289:T7)
            n113 = Not Equal?(x=w289, y=w287) -> (x != y?=w288:bool)
            n114 = case shown="True" w288 {
              tunnel: [w298 w299] -> w294
              tunnel: w291 -> [w297 w299]
              tunnel: w290 -> [w296 _]
              tunnel: w287 -> [w295 _]
              frame True {
                n115 = invoke class="VI" method="FP.Open"(reference=w296, error in=w297, "State"=w295) -> (error out=w298:errorcluster)  [unwired: 2 in, 4 out]
              }
              frame False {
              }
            }
          }
          frame "Minimize", "Minimized" {
            w300 = T7."Minimized" ("State")
            n116 = property class="VI"(reference=w306, error in=w305) -> (reference out=w303:refnum<vi>, error out=w304:errorcluster, "FP.State"=w302:T7)
            n117 = Not Equal?(x=w302, y=w300) -> (x != y?=w301:bool)
            n118 = case shown="True" w301 {
              tunnel: [w311 w312] -> w307
              tunnel: w304 -> [w310 w312]
              tunnel: w303 -> [w309 _]
              tunnel: w300 -> [w308 _]
              frame True {
                n119 = invoke class="VI" method="FP.Open"(reference=w309, error in=w310, "State"=w308) -> (error out=w311:errorcluster)  [unwired: 2 in, 4 out]
              }
              frame False {
              }
            }
          }
          frame "Maximize", "Maximized" {
            w313 = T7."Maximized" ("State")
            n120 = property class="VI"(reference=w319, error in=w318) -> (reference out=w316:refnum<vi>, error out=w317:errorcluster, "FP.State"=w315:T7)
            n121 = Not Equal?(x=w315, y=w313) -> (x != y?=w314:bool)
            n122 = case shown="True" w314 {
              tunnel: [w324 w325] -> w320
              tunnel: w317 -> [w323 w325]
              tunnel: w316 -> [w322 _]
              tunnel: w313 -> [w321 _]
              frame True {
                n123 = invoke class="VI" method="FP.Open"(reference=w322, error in=w323, "State"=w321) -> (error out=w324:errorcluster)  [unwired: 2 in, 4 out]
              }
              frame False {
              }
            }
          }
        }
        n124 = call <vilib>:"Add State(s) to Queue__JKI_lib_State_Machine.vi"("State(s) in (\"\")"=w260) -> ("States Out"=w259:string)  [unwired: 14 in]
      }
      frame "UI: Refresh CSM List" {
        n125 = property on="CSM" class="CmbBox"() -> ("Value"=w329:string)  [unwired: 2 in, 2 out]
        n126 = call <userlib>:"CSM - List Modules.vi"() -> ("error out"=w326:errorcluster, "Module Names"=w331:string[])  [unwired: 10 in]
        n127 = Search 1D Array(1D array=w331, element=w329) -> (index of element=w327:i32)  [unwired: 1 in]
        n128 = Greater Or Equal To 0?(x=w327) -> (x >= 0?=w328:bool)
        n129 = Index Array(array=w331) -> (element=w330:string)  [unwired: 1 in]
        n130 = Select(t=w329, s=w328, f=w330) -> (s? t:f=w332:string)
        n131 = property on="CSM" class="CmbBox"("Strings[]"=w331, "Value"=w332) -> ()  [unwired: 2 in, 2 out]
        n132 = call <vilib>:"Simple Error Handler.vi"("error in (no error)"=w326) -> ()  [unwired: 4 in, 5 out]
      }
      frame "UI: Update Broadcast Registry" {
        n133 = call <userlib>:"CSM - List Rules in Broadcast Registry.vi"() -> ("Rule Entries"=w337:T13)  [unwired: 9 in, 2 out]
        n134 = for {
          tunnel: w337 -> [w349] mode=indexing
          tunnel: [w344] -> w340 mode=indexing
          n135 = Unbundle(w349) -> ("Status"=w348:string, "Source CSM"=w347:string, "Target CSM"=w346:string, "Target API"=w345:string)
          n136 = Build Array(w348, w347, w346, w345) -> (w344:string[])
        }
        "Broadcast Registry" <- w340
        n137 = call <vilib>:"Add State(s) to Queue__JKI_lib_State_Machine.vi"("State(s) in (\"\")"=w338) -> ("States Out"=w339:string)  [unwired: 14 in]
      }
      frame "UI: Update Mermaid" {
        n138 = Unbundle By Name(w356) -> ("Mermaid.string"=w351:string, "Mermaid.Template"=w354:string, "Mermaid.output path"=w355:path)
        "mermaid string" <- w351
        n139 = feedback-in #2(w351) -> ()
        n140 = feedback #2("" ("string")) -> (w352:string)
        n141 = Not Equal?(x=w351, y=w352) -> (x != y?=w350:bool)
        n142 = case shown="True" w350 {
          tunnel: w355 -> [_ w367]
          tunnel: w354 -> [_ w365]
          tunnel: w351 -> [_ w362]
          frame False {
          }
          frame True {
            n143 = Search and Replace String(input string=w365, search string="%s", replace string=w362) -> (result string=w363:string)  [unwired: 5 in, 3 out]
            n144 = Text to UTF-8(11:w363) -> (3:w366:string)  [unwired: 2 in, 1 out]
            n145 = Write to Text File(file (use dialog)=w367, text=w366) -> ()  [unwired: 2 in, 3 out]
            n146 = Path To String(path=w367) -> (string=w361:string)
            n147 = invoke on="WebView2 Control" class="WebView2 Control (strict)" method="Navigate And Wait.vi"("Source"=w361, "Timeout (Inf)"=2000) -> ()  [unwired: 5 in, 7 out]
          }
        }
      }
      frame "UI: Update Toolbar" {
        n148 = Unbundle By Name(w373) -> ("Core.Current VI Reference"=w372:refnum<vi>, "LogFile"=w369:path)  [unwired: 1 out]
        n149 = Empty String/Path?(string/path=w369) -> (empty?=w368:bool)
        n150 = case shown="True" w368 {
          tunnel: "Running Log Viewer (CSM)" ("Front Panel Window:Title") -> [w381 w382]
          tunnel: [w380 w382] -> w370
          tunnel: w369 -> [w377 _]
          frame False {
            n151 = Path To String(path=w377) -> (string=w378:string)
            n152 = Concatenate Strings(w381, " - " ("string"), w378) -> (w380:string)
          }
          frame True {
          }
        }
        n153 = property class="VI"(reference=w372, "Front Panel.Title"=w370) -> ()  [unwired: 1 in, 2 out]
      }
      frame "UI: Resize Tab Content" {
        w393 = u32 16 ("y")
        w389 = 8 ("Position:Left")
        n154 = control-ref of="Tab"() -> (w396:refnum<vi>)
        n155 = invoke class="TabCtl (strict)" method="FitControlToPane"(reference=w396) -> (reference out=w390:refnum<vi>)  [unwired: 2 in, 2 out]
        n156 = control-ref of="WebView2 Control"() -> (w383:refnum<vi>)
        n157 = property class="TabCtl (strict)"(reference=w390) -> ("PaneHeight"=w395:u32, "PaneWidth"=w394:u32, "TabHeight"=w391:u32)  [unwired: 1 in, 2 out]
        n158 = control-ref of="mermaid string"() -> (w384:refnum<vi>)
        n159 = control-ref of="Broadcast Registry"() -> (w392:refnum<vi>)
        n160 = Build Array(w384) -> (w385:refnum<vi>[])
        n161 = Subtract(x=w394, y=w393) -> (x-y=w386:u32)
        n162 = Subtract(x=w395, y=w393) -> (x-y=w387:u32)
        n163 = Add(x=w389, y=w391) -> (x+y=w388:u32)
        n164 = for {
          tunnel: w389 -> [w405]
          tunnel: w388 -> [w404]
          tunnel: w387 -> [w403]
          tunnel: w386 -> [w402]
          tunnel: w385 -> [w401] mode=indexing
          n165 = property class="Str"(reference=w401, "Left"=w405, "Top"=w404, "Height"=w403, "Width"=w402) -> ()  [unwired: 1 in, 2 out]
        }
        n166 = property class="Tbl (strict)"(reference=w392, "Left"=w389, "Top"=w388, "Height"=w387, "Width"=w386) -> ()  [unwired: 1 in, 2 out]
        n167 = property class="WebView2 Control (strict)"(reference=w383, "Left"=w389, "Top"=w388, "Height"=w387, "Width"=w386) -> ()  [unwired: 1 in, 2 out]
      }
      frame "---------- Macro ----------" {
        # "Do not put any code in this frame.\n(It is a separator no-op. You can make a copy of this frame to create a new Macro frame)"
        n168 = call <vilib>:"Add State(s) to Queue__JKI_lib_State_Machine.vi"("State(s) in (\"\")"=w410) -> ("States Out"=w409:string)  [unwired: 14 in]
      }
      frame "Macro: Initialize" {
        w412 = "Data: Initialize\nData: Initialize References\nInitialize Core Data\nUI: Initialize\nUI: Front Panel State >> Open\nUI: Resize Tab Content\nUI: Refresh CSM List\nUI: Update Toolbar\nUI: Update Broadcast Registry\nMermaid: Update Broadcast Registry\nUI: Update Mermaid"  # Data: Initialize Data: Initialize References Initialize Core Data UI: Initialize UI: Front Panel State >> Open UI: Resize Tab Content UI: Refresh CSM List UI: Update Toolbar UI: Update Broadcast Registry Mermaid: Update Broadcast Registry UI: Update Mermaid
        # "Initialization Macro\n(This is called once, when the VI starts)"
        n169 = call <vilib>:"Add State(s) to Queue__JKI_lib_State_Machine.vi"("State(s) in Front (\"\")"=w412, "State(s) in (\"\")"=w416) -> ("States Out"=w415:string)  [unwired: 13 in]
      }
      frame "Macro: Exit" {
        # "Exit Macro\n(This is called once, when the VI exits)"
        n170 = Unbundle By Name(w417) -> ("Core.Close Panel on Exit?"=w429:bool)
        n171 = Unbundle By Name(w417) -> ("Mermaid.output path"=w422:path)
        n172 = call <vilib>:"Check if File or Folder Exists.vi"("path"=w422) -> ("error out"=w421:errorcluster, "file or folder exists?"=w418:bool, "dup path"=w420:path)  [unwired: 8 in]
        n173 = case shown="True" w418 {
          tunnel: w421 -> [w433 w436]
          tunnel: w420 -> [_ w435]
          tunnel: [w433 w434] -> w419
          frame False {
          }
          frame True {
            n174 = Delete(path (use dialog)=w435, error in=w436) -> (error out=w434:errorcluster)  [unwired: 3 in, 2 out]
          }
        }
        n175 = call <vilib>:"Clear Errors.vi"("error in (no error)"=w419) -> ()  [unwired: 5 in, 2 out]
        n176 = Select(t="//UI: Front Panel State >> Close", s=w429, f="") -> (s? t:f=w426:string)
        n177 = call <vilib>:"Add State(s) to Queue__JKI_lib_State_Machine.vi"("State(s) in (\"\")"=w426, "State(s) at Back (\"\")"="Data: Cleanup\nExit") -> ("States Out"=w424:string)  [unwired: 13 in]
        n178 = call <vilib>:"Add State(s) to Queue__JKI_lib_State_Machine.vi"("State(s) in Front (\"\")"=w424, "State(s) in (\"\")"=w432) -> ("States Out"=w431:string)  [unwired: 13 in]
      }
      frame "----------- Mermaid ------------" {
      }
      frame "Mermaid: Update Broadcast Registry" {
        n179 = call "Generate Status-API Mapping mermaid.vi"() -> ("String"=w441:string)  [unwired: 9 in, 2 out]
        n180 = Bundle By Name(cluster=w446, "Mermaid.string"=w441) -> (w444:T10)
        n181 = call <vilib>:"Add State(s) to Queue__JKI_lib_State_Machine.vi"("State(s) in (\"\")"=w442) -> ("States Out"=w443:string)  [unwired: 14 in]
      }
      frame "Mermaid: Update All CSM Interface" {
        n182 = call <userlib>:"CSM - List Modules.vi"() -> ("error out"=w454:errorcluster, "Module Names"=w453:string[])  [unwired: 10 in]
        n183 = for {
          tunnel: [w472] -> w456 mode=indexing if=w466
          tunnel: w455 -> [w471]
          tunnel: w453 -> [w468] mode=indexing
          tunnel: w454 -> [w469]
          n184 = call "Query VIRef with Error Cache.vi"("Current Module(\"\" to generate a ID)"=w471, "Error In (no error)"=w469, "Target Module"=w468) -> ("error out"=w470:errorcluster, "CSM VI Ref"=w461:refnum<vi>)  [unwired: 7 in]
          n185 = call-poly <userlib>:"CSM-Helper API.vi"("error in (no error)"=w470, "VI"=w461) -> ("error out"=w464:errorcluster, "CSM-Helper.lvclass"=w465:refnum<class "CSM-Helper.lvclass">)  [unwired: 8 in]
          n186 = call "Generate CSM Class mermaid(CSMH).vi"("error in (no error)"=w464, "CSM-Helper in"=w465) -> ("error out"=w463:errorcluster, "resulting string"=w472:string, "CSM-Helper out"=w462:refnum<class "CSM-Helper.lvclass">)  [unwired: 7 in]
          n187 = call-poly <userlib>:"CSM-Helper API.vi"("error in (no error)"=w463, "CSM-Helper in"=w462) -> ("error out"=w467:errorcluster)  [unwired: 8 in, 1 out]
          n188 = Not(x=w467) -> (.not. x?=w466:bool)
        }
        n189 = Build Array (concatenate)("classDiagram\ndirection LR", w456) -> (w450:string[])
        n190 = call <userlib>:"1D Array to String_csm.vi"("delimiter (Tab)"="\r", "Array of Strings"=w450) -> ("delimited string"=w452:string)  [unwired: 9 in]
        n191 = Bundle By Name(cluster=w459, "Mermaid.string"=w452) -> (w457:T10)
      }
      frame "Mermaid: Update CSM Interface" {
        n192 = local read "CSM"() -> (w474:string)
        n193 = call "Query VIRef with Error Cache.vi"("Current Module(\"\" to generate a ID)"=w486, "Target Module"=w474) -> ("error out"=w480:errorcluster, "CSM VI Ref"=w473:refnum<vi>)  [unwired: 8 in]
        n194 = call-poly <userlib>:"CSM-Helper API.vi"("error in (no error)"=w480, "VI"=w473) -> ("error out"=w478:errorcluster, "CSM-Helper.lvclass"=w479:refnum<class "CSM-Helper.lvclass">)  [unwired: 8 in]
        n195 = call "Generate CSM Class mermaid(CSMH).vi"("error in (no error)"=w478, "CSM-Helper in"=w479) -> ("error out"=w477:errorcluster, "resulting string"=w487:string, "CSM-Helper out"=w476:refnum<class "CSM-Helper.lvclass">)  [unwired: 7 in]
        n196 = call-poly <userlib>:"CSM-Helper API.vi"("error in (no error)"=w477, "CSM-Helper in"=w476) -> ("error out"=w475:errorcluster)  [unwired: 8 in, 1 out]
        n197 = Build Array("classDiagram\ndirection LR", w487) -> (w483:string[])
        n198 = call <vilib>:"Clear Errors.vi"("error in (no error)"=w475) -> ()  [unwired: 5 in, 2 out]
        n199 = call <userlib>:"1D Array to String_csm.vi"("delimiter (Tab)"="\r", "Array of Strings"=w483) -> ("delimited string"=w485:string)  [unwired: 9 in]
        n200 = Bundle By Name(cluster=w490, "Mermaid.string"=w485) -> (w488:T10)
      }
    }
  }
  n201 = control-ref of="Current VI Reference"() -> (w1:refnum<vi>)
  n202 = call <userlib>:"CSM - Destroy Global Log Event.vi"("Error In"=w5, "CSM Global Log Event"=w11) -> ("error out"=w2:errorcluster)  [unwired: 9 in]
  n203 = call <userlib>:"Close FP if in LabVIEW Dir.vi"("VI Refnum"=w1, "Error in"=w2) -> ("Error out"=w3:errorcluster)  [unwired: 9 in]
  n204 = call <vilib>:"Clear Errors.vi"("error in (no error)"=w3) -> ()  [unwired: 5 in, 2 out]
